vi "Configure Digital Pattern Trigger.vi"(8 "error in (no error)":errorcluster, 9 "Trigger Slope (Positive)":bool=TRUE, 10 "Trigger Source (External)":u16(ring) items=["External", "Bus"], 11 "VISA resource name":refnum<visa-resource-name>) -> (0 "error out":errorcluster, 3 "VISA resource name out":refnum<visa-resource-name>)   [LabVIEW 2017, in "Keithley 3390.lvlib"]
doc: "Configures the Digital Pattern Trigger"
uses:
  Keithley 3390.lvlib
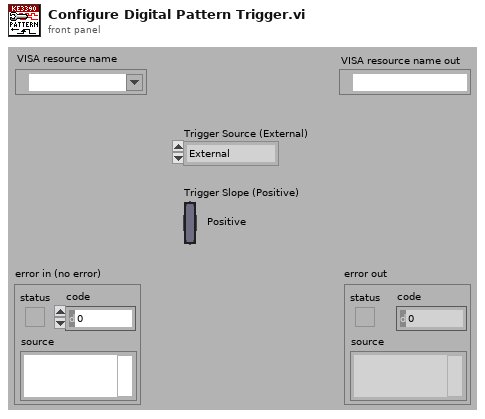
[diagram p1: front panel]
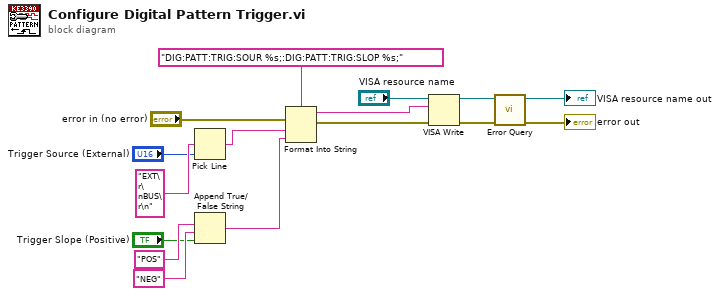
[diagram p0: block diagram]
diagram:
  n1 = Pick Line(multi-line string="EXT\r\nBUS\r\n" ("options"), line index="Trigger Source (External)") -> (output string=w6:string)  [unwired: 1 in]
  n2 = Append True/False String(1:"Trigger Slope (Positive)", 2:"NEG" ("false string"), 3:"POS" ("true string")) -> (0:w5:string)  [unwired: 1 in]
  n3 = Format Into String(format string="DIG:PATT:TRIG:SOUR %s;:DIG:PATT:TRIG:SLOP %s;", error in="error in (no error)", w6, w5) -> (resulting string=w9:string, error out=w8:errorcluster)  [unwired: 1 in]
  n4 = VISA Write(VISA resource name="VISA resource name", write buffer=w9, error in (no error)=w8) -> (VISA resource name out=w3:refnum<visa-resource-name>, error out=w2:errorcluster)  [unwired: 1 out]
  n5 = call "Error Query.vi"("error in (no error)"=w2, "VISA resource name"=w3) -> ("error out"=→"error out":errorcluster, "VISA resource name out"=→"VISA resource name out":refnum<visa-resource-name>)  [unwired: 6 in, 2 out]
